vi "Mappa AI DI PLC_3.vi"(0 "USCITE PLC 2":T1, 1 "MBit read":bool[](array[boolean]), 2 "MW read":dbl[](array[numeric]), 3 "M real read":dbl[](array[numeric]), 4 "Array DB bit":bool[](array[boolean]), 5 "DB WORD":dbl[](array[numeric]), 7 "DB REAL":dbl[](array[numeric])) -> (14 "STATO PLC":T4)   [LabVIEW 2019]
uses:
  STATO PLC 3.ctl
  Uscite PLC 3.ctl
  controls/statoAO_plc_3.ctl
  StatoDO_PLC_3.ctl
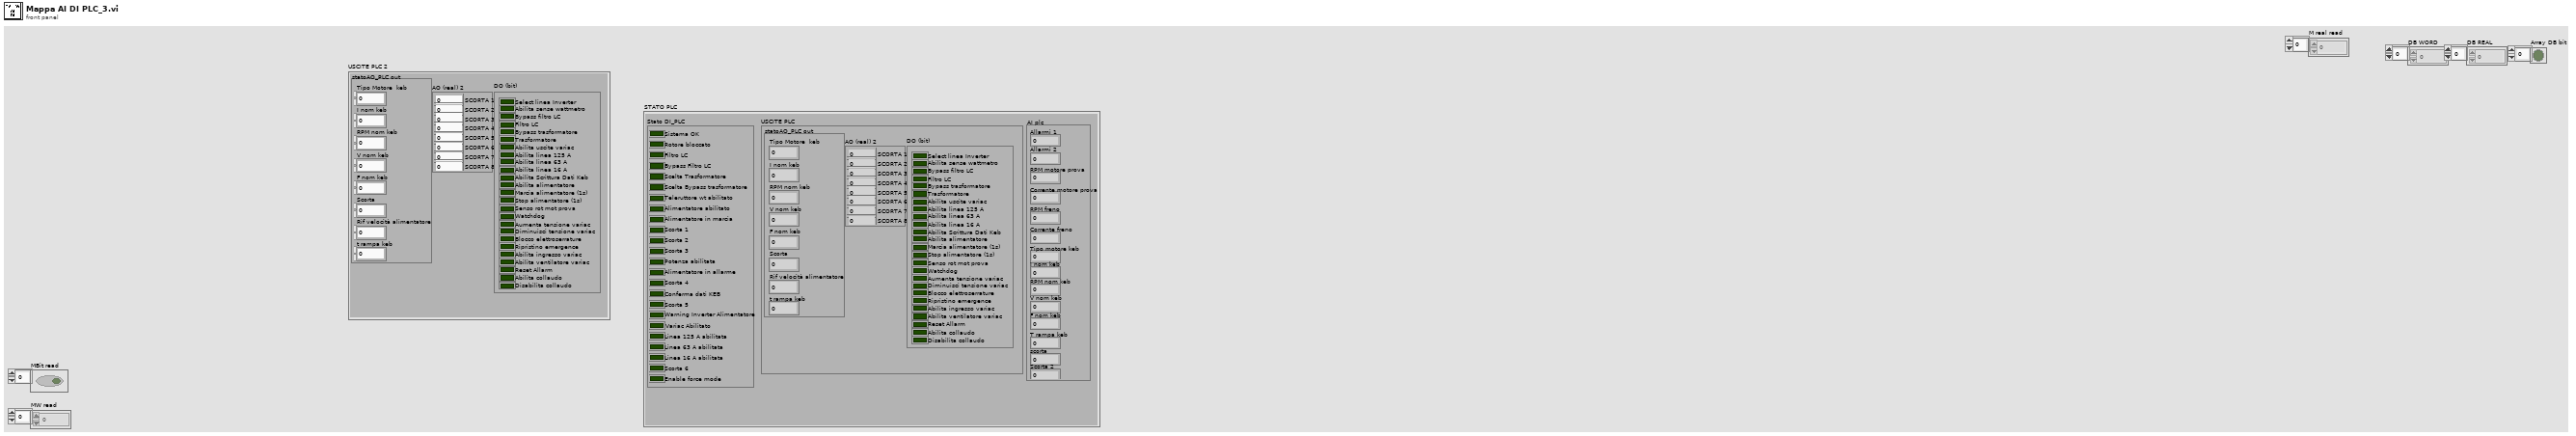
[diagram p1: front panel]
types:
  T1 = typedef "Uscite PLC 3.ctl" = cluster{"AO (real) 2":cluster{"SCORTA 1":dbl, "SCORTA 2":dbl, "SCORTA 3":dbl, "SCORTA 4":dbl, "SCORTA 5":dbl, "SCORTA 6":dbl, "SCORTA 7":dbl, "SCORTA 8":dbl}, "statoAO_PLC out":T2, "DO (bit)":T3}
  T2 = typedef "statoAO_plc_3.ctl" = cluster{"Rif velocità alimentatore":dbl, "Scorta":dbl, "Tipo Motore  keb":dbl, "I nom keb":dbl, "RPM nom keb":dbl, "V nom keb":dbl, "F nom keb":dbl, "t rampa keb":dbl}
  T3 = typedef "StatoDO_PLC_3.ctl" = cluster{"Select linea Inverter":bool, "Abilita sense wattmetro":bool, "Bypass filtro LC":bool, "Filtro LC":bool, "Bypass trasformatore":bool, "Trasformatore":bool, "Abilita uscite variac":bool, "Abilita linea 125 A":bool, "Abilita linea 63 A":bool, "Abilita linea 16 A":bool, "Abilita Scrittura Dati Keb":bool, "Abilita alimentatore":bool, "Marcia alimentatore (1s)":bool, "Stop alimentatore (1s)":bool, "Senso rot mot prova":bool, "Watchdog":bool, "Aumenta tensione variac":bool, "Diminuisci tensione variac ":bool, "Blocco elettroserrature":bool, "Ripristino emergence":bool, "Abilita ingresso variac":bool, "Abilita ventilatore variac":bool, "Reset Allarm":bool, "Scorta 1":bool, "Scorta 2":bool, "Scorta 3":bool, "Scorta 4":bool, "Scorta 5":bool, "Scorta 6":bool, "Scorta 7":bool, "Scorta 8":bool, "Scorta 9":bool, "Abilita collaudo":bool, "Disabilita collaudo ":bool, "Scorta 10":bool, "Scorta 11":bool, "Scorta 12":bool, "Scorta 13":bool, "Scorta 14":bool, "Scorta 15":bool}
  T4 = typedef "STATO PLC 3.ctl" = cluster{"USCITE PLC":T1, "Stato DI_PLC":cluster{"Sistema OK":bool, "Rotore bloccato":bool, "Filtro LC":bool, "Bypass Filtro LC":bool, "Scelta Trasformatore":bool, "Scelta Bypass trasformatore":bool, "Teleruttore wt abilitato":bool, "Alimentatore abilitato":bool, "Alimentatore in marcia":bool, "Scorta 1":bool, "Scorta 2":bool, "Scorta 3":bool, "Potenza abilitata":bool, "Alimentatore in allarme":bool, "Scorta 4":bool, "Conferma dati KEB":bool, "Scorta 5":bool, "Warning Inverter Alimentatore":bool, "Variac Abilitato":bool, "Linea 125 A abilitata":bool, "Linea 63 A abilitata":bool, "Linea 16 A abilitata":bool, "Scorta 6":bool, "Enable force mode":bool}, "AI plc":cluster{"Allarmi 1":dbl, "Allarmi 2":dbl, "RPM motore prova":dbl, "Corrente motore prova":dbl, "RPM freno":dbl, "Corrente freno":dbl, "Tipo motore keb":dbl, "I nom keb":dbl, "RPM nom keb":dbl, "V nom keb":dbl, "F nom keb":dbl, "T rampa keb":dbl, "scorta":dbl, "Scorta 2":dbl}}
  T5 = cluster{"Allarmi 1":dbl, "Allarmi 2":dbl, "RPM motore prova":dbl, "Corrente motore prova":dbl, "RPM freno":dbl, "Corrente freno":dbl, "Tipo motore keb":dbl, "I nom keb":dbl, "RPM nom keb":dbl, "V nom keb":dbl, "F nom keb":dbl, "T rampa keb":dbl, "scorta":dbl, "Scorta 2":dbl}
  T6 = cluster{"MBit read[0]":bool, "MBit read[1]":bool, "MBit read[2]":bool, "MBit read[3]":bool, "MBit read[4]":bool, "MBit read[5]":bool, "MBit read[6]":bool, "MBit read[7]":bool, "MBit read[8]":bool, "MBit read[9]":bool, "MBit read[10]":bool, "MBit read[11]":bool, "MBit read[12]":bool, "MBit read[13]":bool, "MBit read[14]":bool, "MBit read[15]":bool, "MBit read[16]":bool, "MBit read[17]":bool, "MBit read[18]":bool, "MBit read[19]":bool, "MBit read[20]":bool, "MBit read[21]":bool, "MBit read[22]":bool, "MBit read[23]":bool}
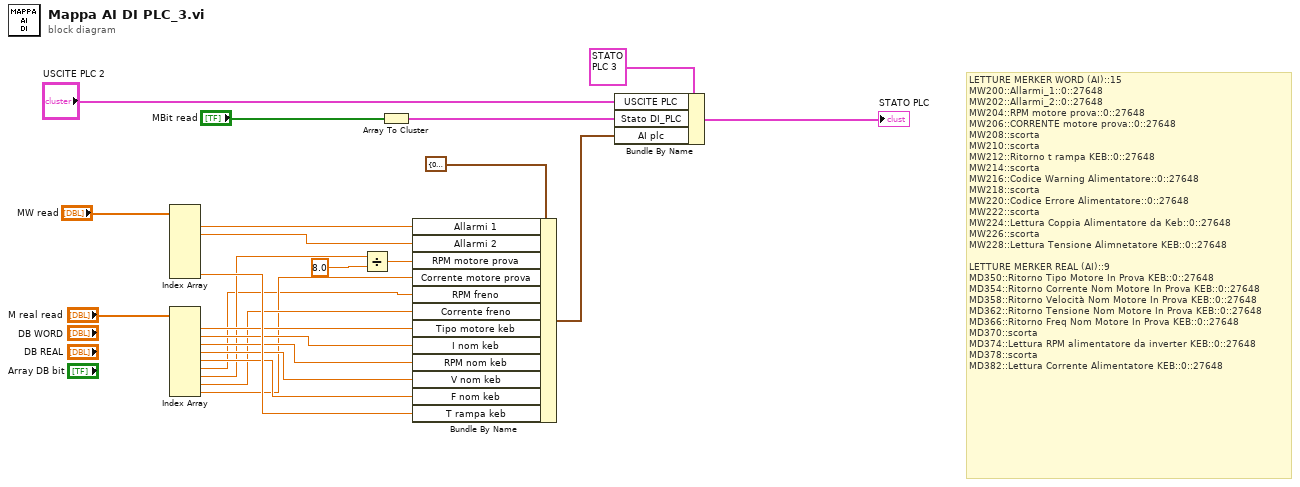
[diagram p0: block diagram]
diagram:
  # "LETTURE MERKER WORD (AI)::15\nMW200::Allarmi_1::0::27648\nMW202::Allarmi_2::0::27648\nMW204::RPM motore prova::0::27648\nMW206::CORRENTE motore prova::0::27648\nMW208::scorta\nMW210::scorta\nMW212::Ritorno t rampa KEB::0::27648\nMW214::scorta\nMW216::Codice Warning Alimentatore::0::27648\nMW218::scorta\nMW220::Codice Errore Alimentatore::0::27648\nMW222::scorta\nMW224::Lettura Coppia Alimentatore da Keb::0::27648\nMW226::scorta\nMW228::Lettura Tensione Alimnetatore KEB::0::27648\n\nLETTURE MERKER REAL (AI)::9\nMD350::Ritorno Tipo Motore In Prova KEB::0::27648\nMD354::Ritorno Corrente Nom Motore In Prova KEB::0::27648\nMD358::Ritorno Velocità Nom Motore In Prova KEB::0::27648\nMD362::Ritorno Tensione Nom Motore In Prova KEB::0::27648\nMD366::Ritorno Freq Nom Motore In Prova KEB::0::27648\nMD370::scorta\nMD374::Lettura RPM alimentatore da inverter KEB::0::27648\nMD378::scorta\nMD382::Lettura Corrente Alimentatore KEB::0::27648"
  n1 = Index Array(array="MW read") -> (element #1=w16:dbl, element #2=w15:dbl, element #7=w14:dbl)  [unwired: 7 in, 4 out]
  n2 = Index Array(array="M real read") -> (element #1=w13:dbl, element #2=w12:dbl, element #3=w11:dbl, element #4=w10:dbl, element #5=w9:dbl, element #6=w1:dbl, element #7=w4:dbl, element #8=w6:dbl, element #9=w5:dbl)  [unwired: 9 in]
  n3 = Divide(x=w4, y=8.0) -> (x/y=w3:dbl)
  n4 = Array To Cluster(array="MBit read") -> (cluster=w22:T6)
  n5 = Bundle By Name(cluster=T5 {"Allarmi 1"=0.0, "Allarmi 2"=0.0, "RPM motore prova"=0.0, "Corrente motore prova"=0.0, "RPM freno"=0.0, "Corrente freno"=0.0, "Tipo motore keb"=0.0, "I nom keb"=0.0, "RPM nom keb"=0.0, "V nom keb"=0.0, "F nom keb"=0.0, "T rampa keb"=0.0, "scorta"=0.0, "Scorta 2"=0.0} ("AI plc"), "Allarmi 1"=w16, "Allarmi 2"=w15, "RPM motore prova"=w3, "Corrente motore prova"=w5, "RPM freno"=w1, "Corrente freno"=w6, "Tipo motore keb"=w13, "I nom keb"=w12, "RPM nom keb"=w11, "V nom keb"=w10, "F nom keb"=w9, "T rampa keb"=w14) -> (w8:T5)
  n6 = Bundle By Name(cluster=T4 {"USCITE PLC"={"AO (real) 2"={"SCORTA 1"=0.0, "SCORTA 2"=0.0, "SCORTA 3"=0.0, "SCORTA 4"=0.0, "SCORTA 5"=0.0, "SCORTA 6"=0.0, "SCORTA 7"=0.0, "SCORTA 8"=0.0}, "statoAO_PLC out"={"Rif velocità alimentatore"=0.0, "Scorta"=0.0, "Tipo Motore  keb"=0.0, "I nom keb"=0.0, "RPM nom keb"=0.0, "V nom keb"=0.0, "F nom keb"=0.0, "t rampa keb"=0.0}, "DO (bit)"={"Select linea Inverter"=FALSE, "Abilita sense wattmetro"=FALSE, "Bypass filtro LC"=FALSE, "Filtro LC"=FALSE, "Bypass trasformatore"=FALSE, "Trasformatore"=FALSE, "Abilita uscite variac"=FALSE, "Abilita linea 125 A"=FALSE, "Abilita linea 63 A"=FALSE, "Abilita linea 16 A"=FALSE, "Abilita Scrittura Dati Keb"=FALSE, "Abilita alimentatore"=FALSE, "Marcia alimentatore (1s)"=FALSE, "Stop alimentatore (1s)"=FALSE, "Senso rot mot prova"=FALSE, "Watchdog"=FALSE, "Aumenta tensione variac"=FALSE, "Diminuisci tensione variac "=FALSE, "Blocco elettroserrature"=FALSE, "Ripristino emergence"=FALSE, "Abilita ingresso variac"=FALSE, "Abilita ventilatore variac"=FALSE, "Reset Allarm"=FALSE, "Scorta 1"=FALSE, "Scorta 2"=FALSE, "Scorta 3"=FALSE, "Scorta 4"=FALSE, "Scorta 5"=FALSE, "Scorta 6"=FALSE, "Scorta 7"=FALSE, "Scorta 8"=FALSE, "Scorta 9"=FALSE, "Abilita collaudo"=FALSE, "Disabilita collaudo "=FALSE, "Scorta 10"=FALSE, "Scorta 11"=FALSE, "Scorta 12"=FALSE, "Scorta 13"=FALSE, "Scorta 14"=FALSE, "Scorta 15"=FALSE}}, "Stato DI_PLC"={"Sistema OK"=FALSE, "Rotore bloccato"=FALSE, "Filtro LC"=FALSE, "Bypass Filtro LC"=FALSE, "Scelta Trasformatore"=FALSE, "Scelta Bypass trasformatore"=FALSE, "Teleruttore wt abilitato"=FALSE, "Alimentatore abilitato"=FALSE, "Alimentatore in marcia"=FALSE, "Scorta 1"=FALSE, "Scorta 2"=FALSE, "Scorta 3"=FALSE, "Potenza abilitata"=FALSE, "Alimentatore in allarme"=FALSE, "Scorta 4"=FALSE, "Conferma dati KEB"=FALSE, "Scorta 5"=FALSE, "Warning Inverter Alimentatore"=FALSE, "Variac Abilitato"=FALSE, "Linea 125 A abilitata"=FALSE, "Linea 63 A abilitata"=FALSE, "Linea 16 A abilitata"=FALSE, "Scorta 6"=FALSE, "Enable force mode"=FALSE}, "AI plc"={"Allarmi 1"=0.0, "Allarmi 2"=0.0, "RPM motore prova"=0.0, "Corrente motore prova"=0.0, "RPM freno"=0.0, "Corrente freno"=0.0, "Tipo motore keb"=0.0, "I nom keb"=0.0, "RPM nom keb"=0.0, "V nom keb"=0.0, "F nom keb"=0.0, "T rampa keb"=0.0, "scorta"=0.0, "Scorta 2"=0.0}} ("STATO PLC"), "USCITE PLC"="USCITE PLC 2", "Stato DI_PLC"=w22, "AI plc"=w8) -> (→"STATO PLC":T4)
